vi "Set Trigger Source Analog Out.vi"(8 "error in (no error)":errorcluster, 9 "trigsrc":T1, 10 "idxChannel":i32, 11 "hdwf":i32) -> (0 "error out":errorcluster, 3 "hdwf out":i32)   [LabVIEW 2014, in "AnalogDiscSDKLv.lvlib"]
doc: "extern \"C\" __declspec(dllexport) int SetTriggerSource_AnalogOut(\n HDWF hdwf,\n int idxChannel,\n TRIGSRC trigsrc\n );"
uses:
  <instrlib>/AnalogDiscSDKLv/AnalogDiscSDKLv.lvlib
  <instrlib>/AnalogDiscSDKLv/AnalogDiscSDKLv.dll
  <instrlib>/AnalogDiscSDKLv/VIs/DWF_TrigSrc.ctl
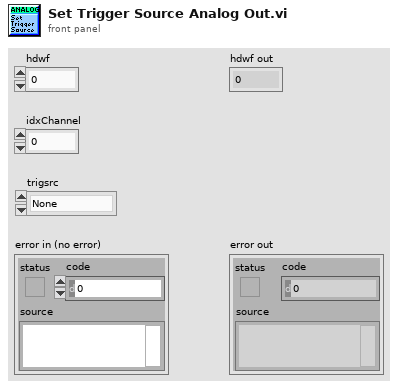
[diagram p1: front panel]
types:
  T1 = typedef "AnalogDiscSDKLv.lvlib/DWF_TrigSrc.ctl" = enum16{"None", "PC", "DetectorAnalogIn", "DetectorDigitalIn", "AnalogIn", "DigitalIn", "DigitalOut", "AnalogOut1", "AnalogOut2", "AnalogOut3", "AnalogOut4", "External1", "External2", "External3", "External4"}
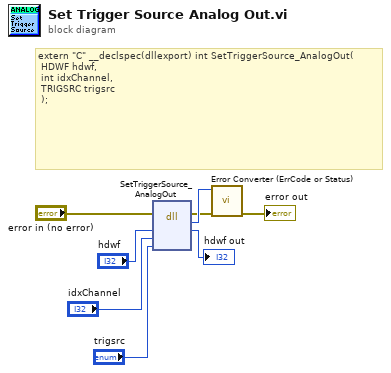
[diagram p0: block diagram]
diagram:
  # "extern \"C\" __declspec(dllexport) int SetTriggerSource_AnalogOut(\n\tHDWF hdwf,\n\tint idxChannel,\n\tTRIGSRC trigsrc\n\t);"
  n1 = dll-call lib="C:/Program Files (x86)/National Instruments/LabVIEW 2014/instr.lib/AnalogDiscSDKLv/AnalogDiscSDKLv.*" fn="SetTriggerSource_AnalogOut"(error in="error in (no error)", "hdwf"="hdwf", "idxChannel"="idxChannel", "trigsrc"="trigsrc") -> (error out=w2:errorcluster, w3:i32, "hdwf"=→"hdwf out":i32)  [unwired: 4 in, 1 out]
  n2 = call <instrlib>:"Error Converter (ErrCode or Status).vi"("error in (no error)"=w2, "error code"=w3) -> ("error out"=→"error out":errorcluster)  [unwired: 9 in]
